vi "Generate Get Connections Error Message.vi"(6 "pin type":T1, 8 "error in":errorcluster, 9 "instrument type id":string, 10 "site":i32, 11 "pin or relay names":string) -> (0 "error out":errorcluster, 3 "error string":string)   [LabVIEW 2020, in "Measurement Plugin Session Management V1.lvlib" / "Session Reservation.lvclass"]
uses:
  Session Reservation.lvclass
  Pin Type.ctl
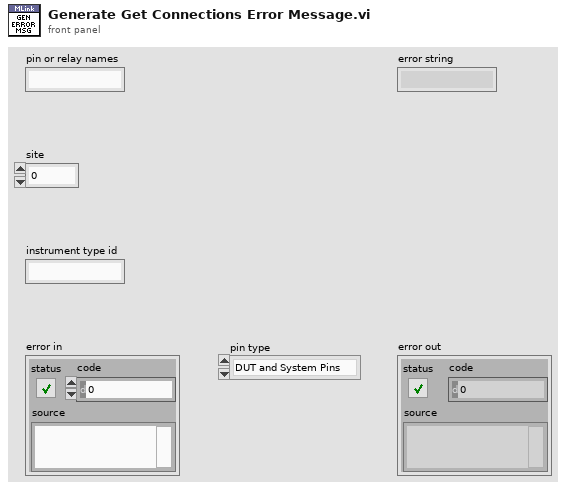
[diagram p1: front panel]
types:
  T1 = typedef "Measurement Plugin Session Management V1.lvlib/Session Reservation.lvclass/Pin Type.ctl" = enum16{"DUT and System Pins", "System Pins"}
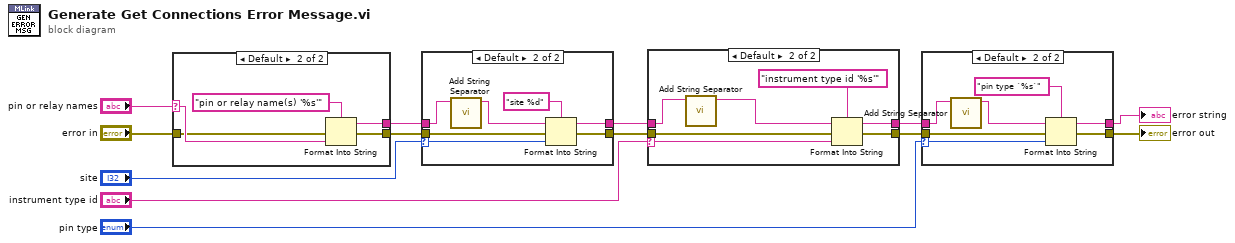
[diagram p0: block diagram]
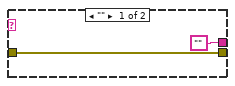
[diagram p3: hidden frame]
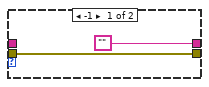
[diagram p5: hidden frame]
diagram:
  n1 = case shown="Default" "pin or relay names" {
    selector: "pin or relay names" -> [_ w18]
    tunnel: ["" w20] -> w11
    tunnel: "error in" -> [w14 w17]
    tunnel: [w14 w16] -> w12
    frame "" {
    }
    frame Default {
      n2 = Format Into String(format string="pin or relay name(s) '%s'", error in=w17, w18) -> (resulting string=w20:string, error out=w16:errorcluster)  [unwired: 1 in]
    }
  }
  n3 = case shown="Default" "site" {
    selector: "site" -> [_ w27]
    tunnel: ["" w29] -> w8
    tunnel: w12 -> [w21 w26]
    tunnel: [w21 w25] -> w6
    tunnel: w11 -> [_ w24]
    frame -1 {
    }
    frame Default {
      n4 = call "Add String Separator.vi"("string in"=w24) -> ("string out"=w23:string)  [unwired: 10 in]
      n5 = Format Into String(format string="site %d", initial string=w23, error in=w26, w27) -> (resulting string=w29:string, error out=w25:errorcluster)
    }
  }
  n6 = case shown="Default" "instrument type id" {
    selector: "instrument type id" -> [_ w34]
    tunnel: [w30 w38] -> w5
    tunnel: w6 -> [w31 w36]
    tunnel: [w31 w35] -> w4
    tunnel: w8 -> [w30 w32]
    frame "" {
    }
    frame Default {
      n7 = call "Add String Separator.vi"("string in"=w32) -> ("string out"=w33:string)  [unwired: 10 in]
      n8 = Format Into String(format string="instrument type id '%s'", initial string=w33, error in=w36, w34) -> (resulting string=w38:string, error out=w35:errorcluster)
    }
  }
  n9 = case shown="Default" "pin type" {
    selector: "pin type" -> [_ w45]
    tunnel: [w39 w47] -> w2
    tunnel: w4 -> [w40 w44]
    tunnel: [w40 w43] -> w1
    tunnel: w5 -> [w39 w42]
    frame "DUT and System Pins" {
    }
    frame Default {
      n10 = call "Add String Separator.vi"("string in"=w42) -> ("string out"=w41:string)  [unwired: 10 in]
      n11 = Format Into String(format string="pin type `%s`", initial string=w41, error in=w44, w45) -> (resulting string=w47:string, error out=w43:errorcluster)
    }
  }
  "error string" <- w2
  "error out" <- w1
